vi "Get days from 1900 and ms since midnight for SAP name.vi"(10 "current time":timestamp) -> (2 "sap filename without id":string)   [LabVIEW 2017]
panel:
  out "ms since midnight":i32
  out "Days Elapsed":i32
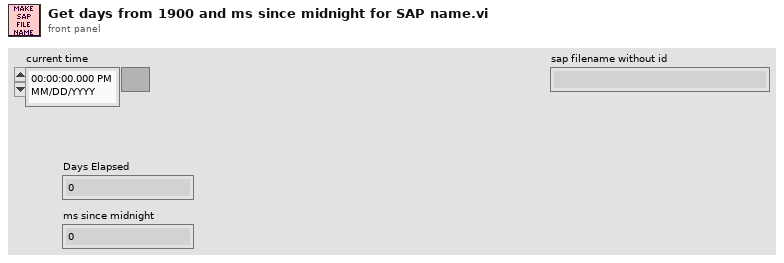
[diagram p1: front panel]
types:
  T1 = typedef "LVDateTimeRec.ctl" = cluster{"fractional second":dbl, "second":i32, "minute":i32, "hour":i32, "day of month":i32, "month":i32, "year":i32, "day of week":i32, "day of year":i32, "DST":i32}
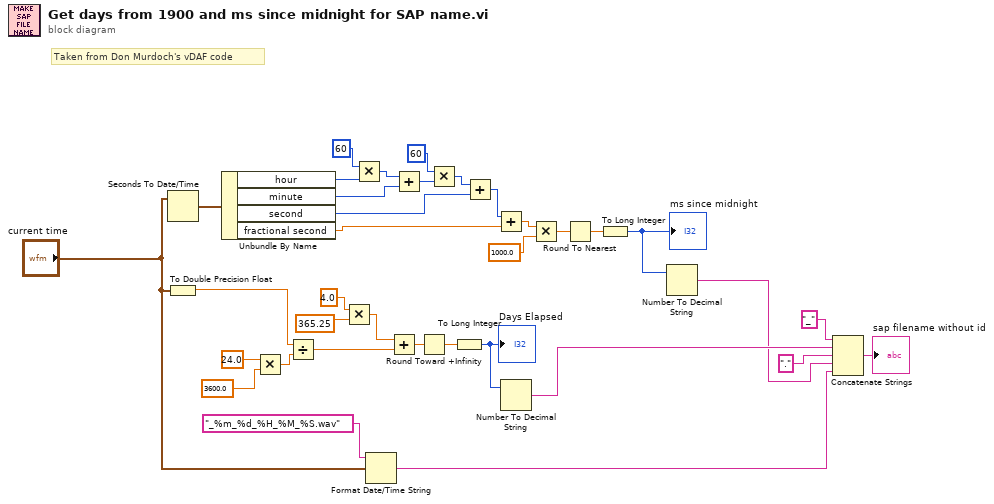
[diagram p0: block diagram]
diagram:
  # "Taken from Don Murdoch's vDAF code"
  n1 = Seconds To Date/Time(time stamp (now)="current time") -> (date time rec=w26:T1)  [unwired: 1 in]
  n2 = To Double Precision Float(number="current time") -> (double precision float=w35:dbl)
  n3 = Unbundle By Name(w26) -> ("hour"=w25:i32, "minute"=w22:i32, "second"=w18:i32, "fractional second"=w17:dbl)
  n4 = Multiply(x=24.0, y=3600.0) -> (x*y=w31:dbl)
  n5 = Divide(x=w35, y=w31) -> (x/y=w32:dbl)
  n6 = Multiply(x=4.0, y=365.25) -> (x*y=w28:dbl)
  n7 = Multiply(x=60, y=w25) -> (x*y=w23:i32)
  n8 = Format Date/Time String(time format string (%c)="_%m_%d_%H_%M_%S.wav", seconds (now)="current time") -> (date/time string=w3:string)  [unwired: 1 in]
  n9 = Add(x=w28, y=w32) -> (x+y=w29:dbl)
  n10 = Add(x=w23, y=w22) -> (x+y=w20:i32)
  n11 = Round Toward +Infinity(x=w29) -> (ceil(x): smallest int >= x=w11:dbl)
  n12 = Multiply(x=60, y=w20) -> (x*y=w19:i32)
  n13 = To Long Integer(number=w11) -> (32bit integer=w8:i32)
  "Days Elapsed" <- w8
  n14 = Add(x=w19, y=w18) -> (x+y=w16:i32)
  n15 = Add(x=w16, y=w17) -> (x+y=w15:dbl)
  n16 = Number To Decimal String(number=w8) -> (decimal integer string=w6:string)  [unwired: 1 in]
  n17 = Multiply(x=w15, y=1000.0) -> (x*y=w13:dbl)
  n18 = Round To Nearest(number=w13) -> (nearest integer value=w12:dbl)
  n19 = To Long Integer(number=w12) -> (32bit integer=w9:i32)
  "ms since midnight" <- w9
  n20 = Number To Decimal String(number=w9) -> (decimal integer string=w4:string)  [unwired: 1 in]
  n21 = Concatenate Strings("_" ("string"), w6, "." ("string"), w4, w3) -> (→"sap filename without id":string)
